vi "No_Change.vi"(9 "Field and Temp Range":T1={"VISA (Magnet)"="COM4", "Fields(T)"=[], "Temps(K)"=[], "VISA (Temp) "="COM1", "Port number (3364)"=3364}, 10 "ScanQ in":refnum<queue>, 11 "Queue in":refnum<queue>) -> (2 "ScanQ out":refnum<queue>, 3 "Queue out":refnum<queue>)   [LabVIEW 2025]
uses:
  Mag & Temp STM/CTLS/Sweeper.ctl
  Mag & Temp STM/CTLS/Scan_Params (QMH).ctl
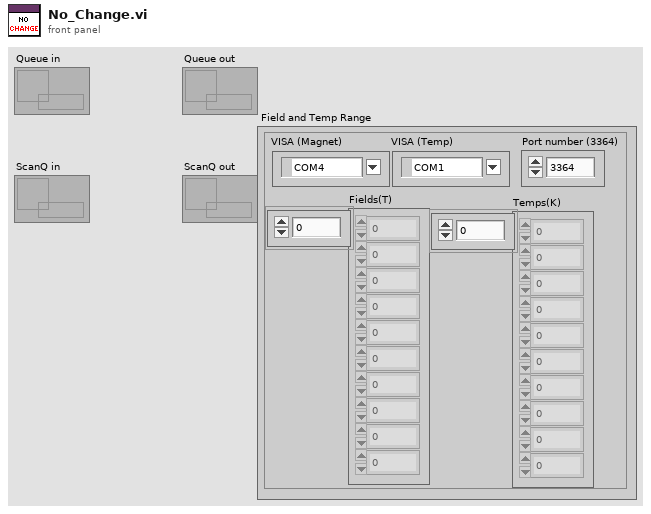
[diagram p1: front panel]
types:
  T1 = cluster{"VISA (Magnet)":refnum<visa-resource-name>, "Fields(T)":dbl[], "Temps(K)":dbl[], "VISA (Temp) ":refnum<visa-resource-name>, "Port number (3364)":u32}
  T2 = enum16{"1. BIAS", "2. INIT_SCAN", "3. SCAN_IDLE", "4. INTER_SCAN", "5. NEW_COORDS_&_FRAME", "6. FINAL_SCAN", "7. POLL BIAS ", "8. Z-CONT.", "9. STOP"}
  T3 = typedef "Scan_Params (QMH).ctl" = cluster{"Setpoint (I)":dbl[], "Bias (V)":dbl[], "Number of scans":u8, "Port number (3364)":u32, "Avoid zero threshold (V)":dbl, "Current State":enum16{"1. BIAS", "2. POLL BIAS", "3. SCAN", "4. SCAN_IDLE", "5. Drift_Correct (SF)", "6. Drift_Correct (BS)", "7. STOP"}}
  T4 = enum16{"NO CHANGE", "SET TEMP & FIELD", "SWEEP IDLE", "NEXT TEMP & FIELD", "SWEEP DONE"}
  T5 = typedef "Sweeper.ctl" = cluster{"Temps(K)":dbl[], "Fields(T)":dbl[], "Sweep States":enum16{"1. Idle", "2. Start", "3. Apply_Config", "4. Run_Point_Step", "5. Wait ACK", "6. Next Field", "7. Next Temp", "8. Stop"}, "PointStep":enum16{"1. Scan_1", "2. DC_SF_1", "3. DC_BS_1", "4. Bias", "5. Scan_2", "6. DC_SF_2", "7. DC_BS_2", "8. Done"}, "Current Field":dbl, "Current Temp":dbl, "Expected_ACK":enum16{"1. None", "2. TempStable", "3. FieldStable", "4. ConfigApplied", "5. ScanDone", "6. BiasDone", "7. DriftDone (SF)", "8. DrifDone (BS)", "9. Done"}, "ACK":enum16{"1. None", "2. TempStable", "3. FieldStable", "4. ConfigApplied", "5. ScanDone", "6. BiasDone", "7. DriftDone (SF)", "8. DrifDone (BS)", "9. Done"}, "AfterAckStep":enum16{"1. Idle", "2. Start", "3. Apply_Config", "4. Run_Point_Step", "5. Wait ACK", "6. Next Field", "7. Next Temp", "8. Stop"}, "Current Index Field":i32, "Current Index Temp":i32, "ACK Structure ":enum16{"Inner", "Outer"}}
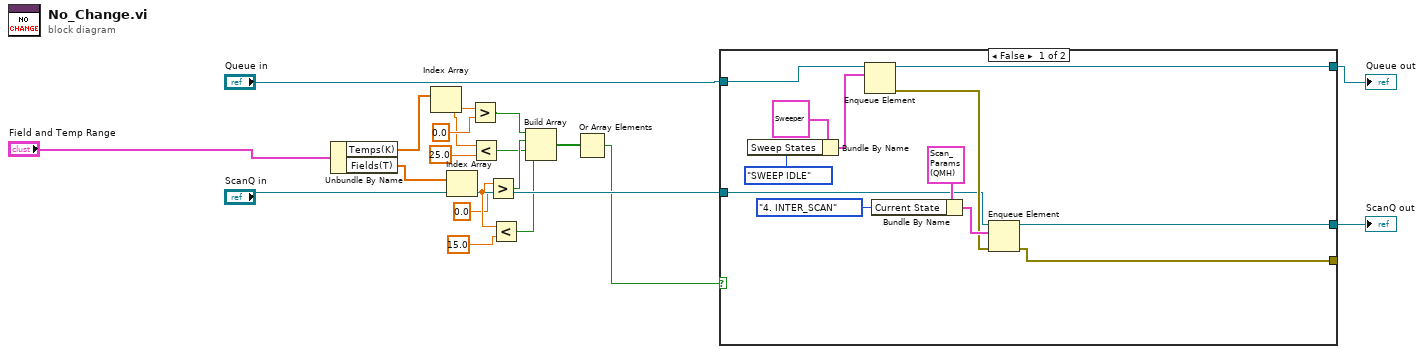
[diagram p0: block diagram]
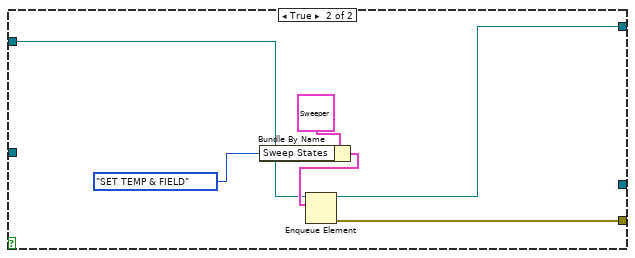
[diagram p2: hidden frame]
diagram:
  n1 = Unbundle By Name("Field and Temp Range") -> ("Temps(K)"=w8:dbl[], "Fields(T)"=w7:dbl[])
  n2 = Index Array(array=w8) -> (element=w2:dbl)  [unwired: 1 in]
  n3 = Index Array(array=w7) -> (element=w13:dbl)  [unwired: 1 in]
  n4 = Greater?(x=w2, y=0.0) -> (0:w5:bool)
  n5 = Less?(x=w2, y=25.0) -> (x < y?=w3:bool)
  n6 = Greater?(x=w13, y=0.0) -> (0:w10:bool)
  n7 = Less?(x=w13, y=15.0) -> (x < y?=w15:bool)
  n8 = Build Array(w5, w10, w3, w15) -> (w12:bool[])
  n9 = Or Array Elements(Boolean array=w12) -> (logical OR=w11:bool)
  n10 = case shown="False" w11 {
    tunnel: [w25 w35] -> w18
    tunnel: [w23 w34] -> _
    tunnel: [w26 _] -> w19
    tunnel: "Queue in" -> [w22 w32]
    tunnel: "ScanQ in" -> [w21 _]
    frame False {
      n11 = Bundle By Name(cluster=T5 {"Temps(K)"=[], "Fields(T)"=[], "Sweep States"=enum."2. Start", "PointStep"=enum."1. Scan_1", "Current Field"=0.0, "Current Temp"=0.0, "Expected_ACK"=enum."1. None", "ACK"=enum."1. None", "AfterAckStep"=enum."1. Idle", "Current Index Field"=-1, "Current Index Temp"=-1, "ACK Structure "=enum."Inner"} ("element"), "Sweep States"=T4."SWEEP IDLE") -> (w29:T5)
      n12 = Enqueue Element(queue=w22, element=w29) -> (queue out=w25:refnum<queue>, error out=w24:errorcluster)  [unwired: 2 in, 1 out]
      n13 = Bundle By Name(cluster=T3 {"Setpoint (I)"=[], "Bias (V)"=[], "Number of scans"=1, "Port number (3364)"=3364, "Avoid zero threshold (V)"=0.004999999888241291, "Current State"=enum."1. BIAS"} ("element"), "Current State"=T2."4. INTER_SCAN") -> (w27:T3)
      n14 = Enqueue Element(queue=w21, element=w27, error in (no error)=w24) -> (queue out=w26:refnum<queue>, error out=w23:errorcluster)  [unwired: 1 in, 1 out]
    }
    frame True {
      n15 = Bundle By Name(cluster=T5 {"Temps(K)"=[], "Fields(T)"=[], "Sweep States"=enum."2. Start", "PointStep"=enum."1. Scan_1", "Current Field"=0.0, "Current Temp"=0.0, "Expected_ACK"=enum."1. None", "ACK"=enum."1. None", "AfterAckStep"=enum."1. Idle", "Current Index Field"=-1, "Current Index Temp"=-1, "ACK Structure "=enum."Inner"} ("element"), "Sweep States"=T4."SET TEMP & FIELD") -> (w36:T5)
      n16 = Enqueue Element(queue=w32, element=w36) -> (queue out=w35:refnum<queue>, error out=w34:errorcluster)  [unwired: 2 in, 1 out]
    }
  }
  "ScanQ out" <- w19
  "Queue out" <- w18
